vi "Write Certificate.vi"(8 "error in (no error)":errorcluster, 10 "Certificate":u8[](array[numeric]), 11 "WebSocket Client in":refnum<class "WebSocket Client.lvclass">) -> (0 "error out":errorcluster, 3 "WebSocket Client out":refnum<class "WebSocket Client.lvclass">)   [LabVIEW 2021, in "WebSocket Actors.lvlib" / "WebSocket Client.lvclass"]
uses:
  WebSocket Client.lvclass
  WebSocket Client.lvclass/WebSocket Client.ctl
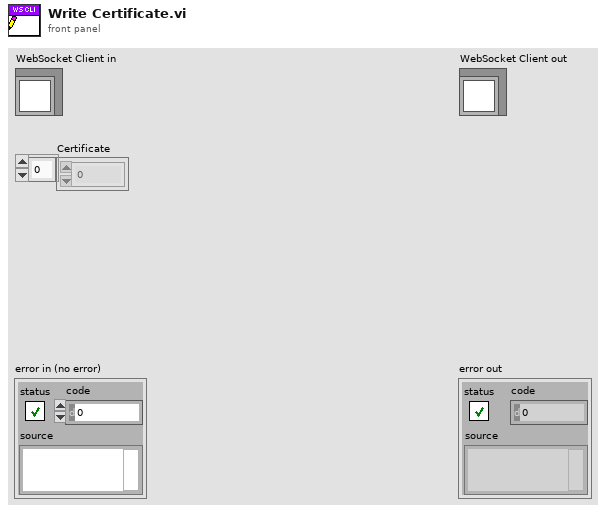
[diagram p1: front panel]
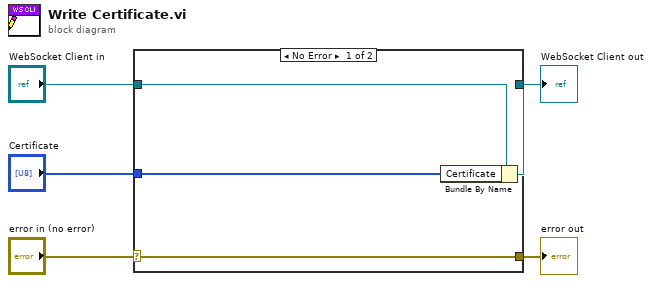
[diagram p0: block diagram]
diagram:
  n1 = case shown="No Error" "error in (no error)" {
    selector: "error in (no error)" -> [w9 w10]
    tunnel: [w9 w10] -> w4
    tunnel: [w7 w11] -> w2
    tunnel: "WebSocket Client in" -> [w8 w11]
    tunnel: "Certificate" -> [w6 _]
    frame No Error {
      n2 = Bundle By Name(cluster=w8, "Certificate"=w6) -> (w7:refnum<class "WebSocket Client.lvclass">)
    }
    frame Error {
    }
  }
  "error out" <- w4
  "WebSocket Client out" <- w2
